vi "Stop Core.vi"(10 "final error code":i32, 11 "Create Project View in":refnum<class "Edit Project View.lvclass">) -> (3 "Create Project View out":refnum<class "Edit Project View.lvclass">)   [LabVIEW 2013, in "Edit Project View.lvlib" / "Edit Project View.lvclass"]
doc: "(<B>Filename</B>: Actor Framework.lvlib:Actor.lvclass:Stop Core.vi)\n\nDefines what the actor does before it stops. Use the <B>final error code</B> input to determine whether the actor shut down in response to an error.\n\nBy default, this method does nothing. A descendant class may override it to define behavior, such as shutting down any processes the actor initiated in its override of the Actor Core method."
uses:
  Edit Project View.lvclass
  <vilib>/ActorFrameworkMVC/View Actor/View Actor.lvclass
  Edit Project View.lvclass/Edit Project View.ctl
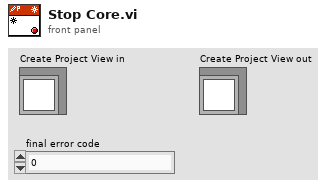
[diagram p1: front panel]
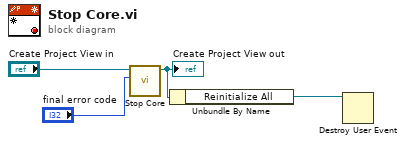
[diagram p0: block diagram]
diagram:
  n1 = call-parent "Stop Core.vi"("final error code"="final error code", "Actor in"="Create Project View in") -> ("Actor out"=w2:refnum<class "Edit Project View.lvclass">)  [unwired: 9 in]
  "Create Project View out" <- w2
  n2 = Unbundle By Name(w2) -> ("Reinitialize All"=w1:refnum<user-event>)
  n3 = Destroy User Event(user event=w1) -> ()  [unwired: 1 in, 1 out]
